vi "extract_pressure.vi"(6 "name":string="AIN0", 7 "R":dbl=283.3, 8 "name_array":string[](array[string]), 9 "value_array":dbl[](array[numeric]), 11 "time":timestamp) -> (0 "P":dbl, 1 "I":dbl, 2 "V":dbl, 3 "waveform_array":waveform(dbl)[](array[waveform])=[{"t0"=timestamp(0 s since 1904-01-01), "dt"=1.0, "Y"=[]}, {"t0"=timestamp(3732035173.078092 s since 1904-01-01), "dt"=1.0, "Y"=[302.8589782714844], "attributes"=variant("NI_ChannelName"=variant(string "T1"))}])   [LabVIEW 2019]
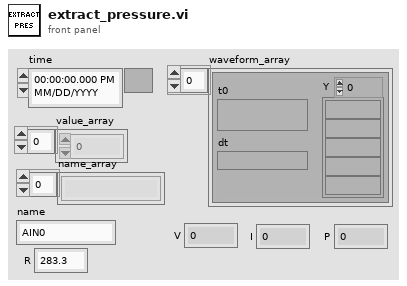
[diagram p1: front panel]
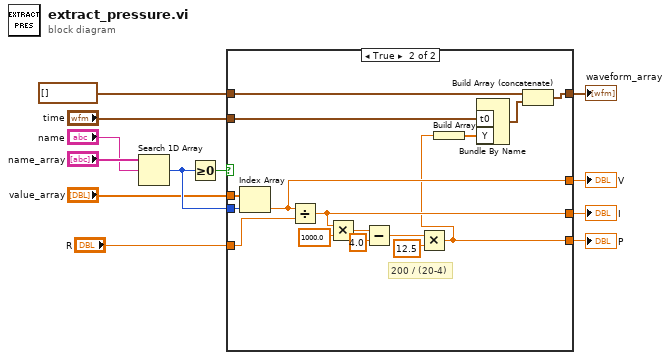
[diagram p0: block diagram]
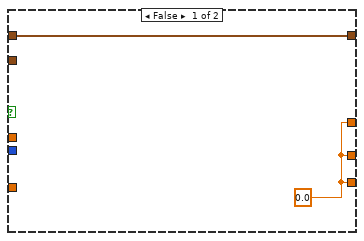
[diagram p2: hidden frame]
diagram:
  n1 = Search 1D Array(1D array="name_array", element="name") -> (index of element=w9:i32)  [unwired: 1 in]
  n2 = Greater Or Equal To 0?(x=w9) -> (x >= 0?=w10:bool)
  n3 = case shown="True" w10 {
    tunnel: w9 -> [_ w30]
    tunnel: "value_array" -> [_ w29]
    tunnel: waveform(dbl)[] [] -> [w14 w28]
    tunnel: "time" -> [_ w27]
    tunnel: [w14 w26] -> w5
    tunnel: [w13 w15] -> w4
    tunnel: [w13 w23] -> w3
    tunnel: "R" -> [_ w22]
    tunnel: [w13 w21] -> w1
    frame False {
      w13 = 0.0 ("CJC (K)")
    }
    frame True {
      # "200 / (20-4)"
      n4 = Index Array(array=w29, index=w30) -> (element=w23:dbl)
      n5 = Divide(x=w23, y=w22) -> (x/y=w21:dbl)
      n6 = Multiply(x=w21, y=1000.0) -> (x*y=w19:dbl)
      n7 = Subtract(x=w19, y=4.0) -> (x-y=w17:dbl)
      n8 = Multiply(x=w17, y=12.5) -> (x*y=w15:dbl)
      n9 = Build Array(w15) -> (w25:dbl[])
      n10 = Bundle By Name("t0"=w27, "Y"=w25) -> (w24:waveform(dbl))  [unwired: 1 in]
      n11 = Build Array (concatenate)(w28, w24) -> (w26:waveform(dbl)[])
    }
  }
  "waveform_array" <- w5
  "P" <- w4
  "V" <- w3
  "I" <- w1
